vi "4080_configure.vi"() -> ()   [LabVIEW 2010]
panel:
  in  "Port Name":string="MainNetwork"
  in  "Frquency Gate Time":bool
  in  "Counter Mode":u16(ring) items=["Pulse Counter", "Frequency"]
  in  "Use checksum":bool
  in  "Baud Rate (9600)":u16(ring)=3 items=["1200 bps", "2400 bps", "4800 bps", "9600 bps", "19.2 kbps", "38.4 kbps"]
  out "Reply":string
  in  "Cheksum":bool
  out "Config String":string
  in  "New Address":u8
  in  "Old Address":u8
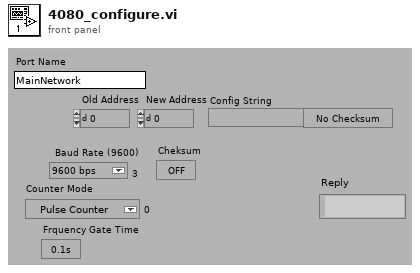
[diagram p1: front panel]
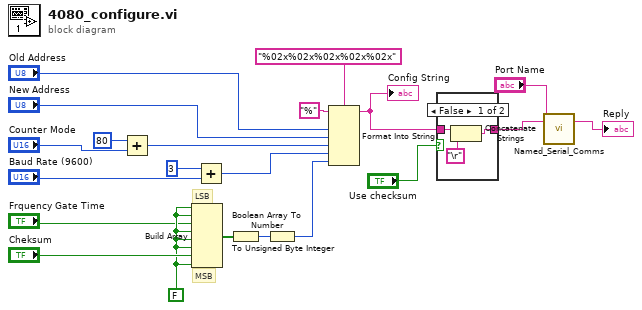
[diagram p0: block diagram]
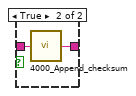
[diagram p2: hidden frame]
diagram:
  w5 = FALSE
  # "MSB"
  # "LSB"
  n1 = Add(x=u16 80, y="Counter Mode") -> (x+y=w6:u16)
  n2 = Build Array(w5, w5, "Frquency Gate Time", w5, w5, w5, "Cheksum", w5) -> (w17:bool[])
  n3 = Add(x=u16 3, y="Baud Rate (9600)") -> (x+y=w11:u16)
  n4 = Boolean Array To Number(Boolean array=w17) -> (number=w15:u32)
  n5 = To Unsigned Byte Integer(number=w15) -> (unsigned 8bit integer=w14:u8)
  n6 = Format Into String(format string="%02x%02x%02x%02x%02x", initial string="%", "Old Address", "New Address", w6, w11, w14) -> (resulting string=w13:string)  [unwired: 1 in, 1 out]
  "Config String" <- w13
  n7 = case shown="False" "Use checksum" {
    tunnel: w13 -> [w24 w26]
    tunnel: [w23 w25] -> w3
    frame False {
      n8 = Concatenate Strings(w24, "\r") -> (w23:string)
    }
    frame True {
      n9 = call "4000_Append_checksum.vi"("ADAM command"=w26) -> ("ADAM string to send"=w25:string)
    }
  }
  n10 = call "Named_Serial_Comms.vi"("Write String"=w3, "Port Name"="Port Name") -> ("Read"=→"Reply":string)  [unwired: 10 in, 3 out]
